vi "requireDataFromPort.vi"(3 "error in (no error)":errorcluster, 4 "Command":string, 5 "VISA resource name":refnum<visa-resource-name>="COM1" caption="端口号") -> (0 "error out":errorcluster, 1 "Data":string, 2 "VISA resource name 2":refnum<visa-resource-name>="COM1" caption="端口号")   [LabVIEW 2010]
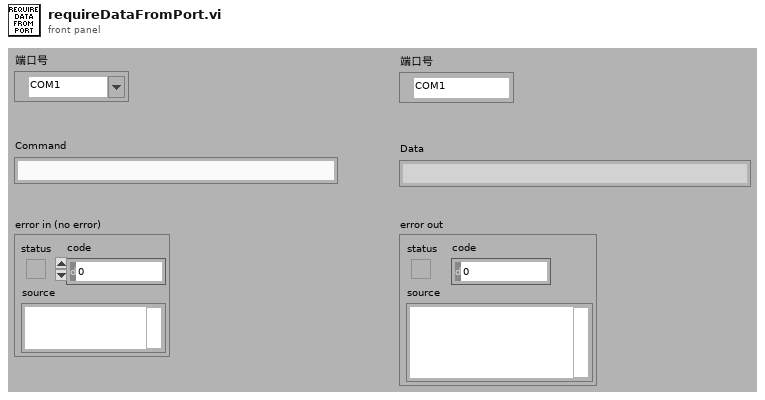
[diagram p1: front panel]
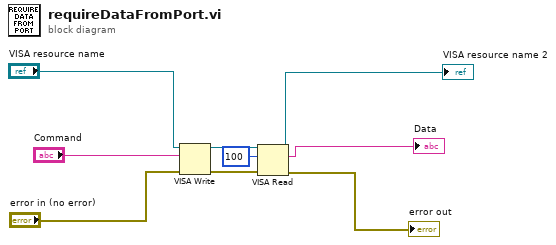
[diagram p0: block diagram]
diagram:
  n1 = VISA Write(VISA resource name="VISA resource name", write buffer="Command", error in (no error)="error in (no error)") -> (VISA resource name out=w9:refnum<visa-resource-name>, error out=w8:errorcluster)  [unwired: 1 out]
  n2 = VISA Read(VISA resource name=w9, byte count=u32 100 ("字节总数"), error in (no error)=w8) -> (VISA resource name out=→"VISA resource name 2":refnum<visa-resource-name>, read buffer=→"Data":string, error out=→"error out":errorcluster)  [unwired: 1 out]
